vi "demo.vi"() -> ()   [LabVIEW 2020]
uses:
  eagle/eagle.lvclass
  Hummingbird/Hummingbird.lvclass
  sheep/sheep.lvclass
  tiger/tiger.lvclass
  Animal/Animal.lvclass
panel:
  out "数组":string[](array[string])
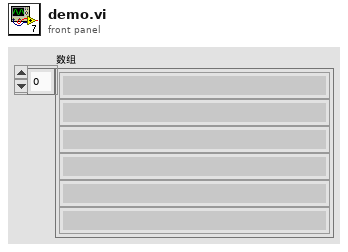
[diagram p1: front panel]
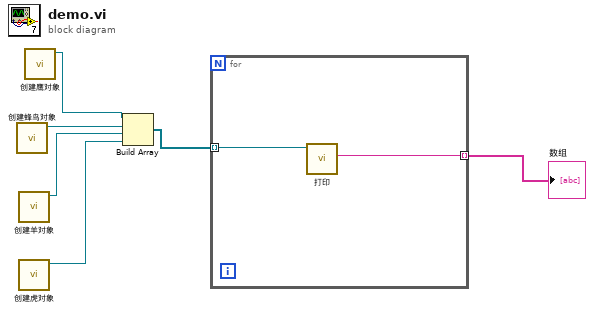
[diagram p0: block diagram]
diagram:
  n1 = call "创建蜂鸟对象.vi"() -> ("Hummingbird.lvclass"=w5:refnum<class "Hummingbird.lvclass">)  [unwired: 11 in]
  n2 = call "创建羊对象.vi"() -> ("Animal输出"=w4:refnum<class "sheep.lvclass">)  [unwired: 11 in]
  n3 = call "创建虎对象.vi"() -> ("Animal输出"=w3:refnum<class "tiger.lvclass">)  [unwired: 11 in]
  n4 = call "创建鹰对象.vi"() -> ("eagle.lvclass"=w6:refnum<class "eagle.lvclass">)  [unwired: 11 in]
  n5 = Build Array(w6, w5, w4, w3) -> (w2:refnum<class "Animal.lvclass">[])
  n6 = for {
    tunnel: w2 -> [w8] mode=indexing
    tunnel: [w7] -> w1 mode=indexing
    n7 = call-dynamic "打印.vi"("Animal 输入"=w8) -> ("字符串"=w7:string)  [unwired: 8 in, 2 out]
  }
  "数组" <- w1
